vi "IHM_errorManagement.vi"(4 "error out":errorcluster, 6 "Cas no error":T1, 7 "No error Line":string) -> (0 "entrée d'erreur (pas d'erreur)":errorcluster, 2 "Cas IHM":T1, 3 "New line Out":string)   [LabVIEW 2009]
uses:
  Commands/IHM_cases.ctl
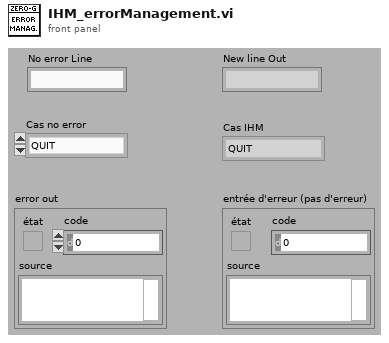
[diagram p1: front panel]
types:
  T1 = typedef "IHM_cases.ctl" = enum16{"QUIT", "INIT IHM", "LOAD CONFIGURATION FILE", "INIT INSTRU", "IHM PROCESS", "CLOSE INSTRU"}
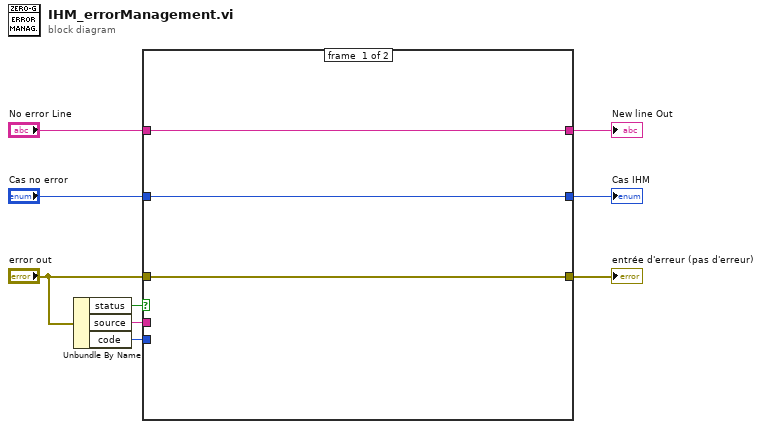
[diagram p0: block diagram]
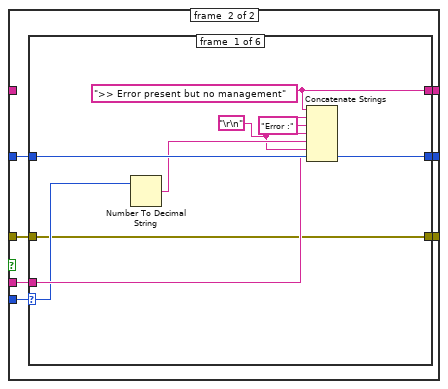
[diagram p2: hidden frame]
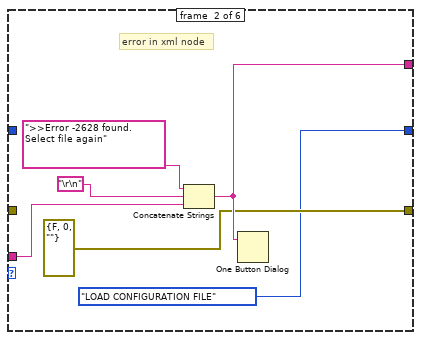
[diagram p3: hidden frame]
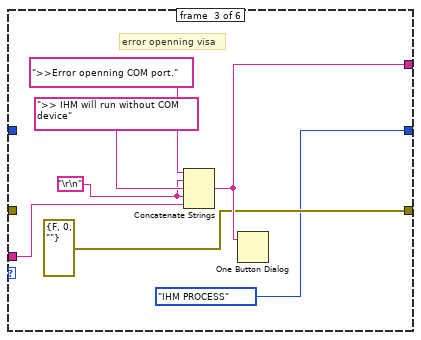
[diagram p4: hidden frame]
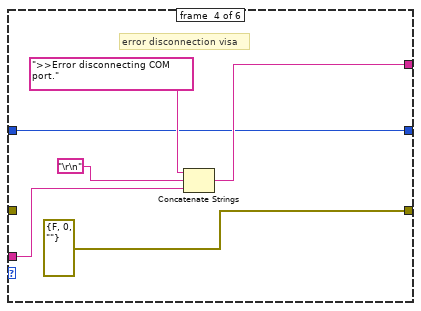
[diagram p5: hidden frame]
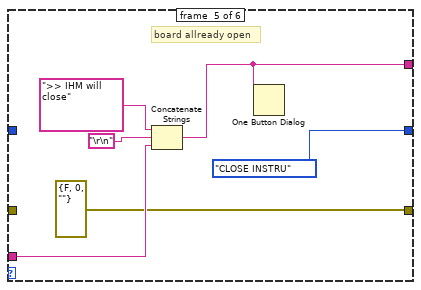
[diagram p6: hidden frame]
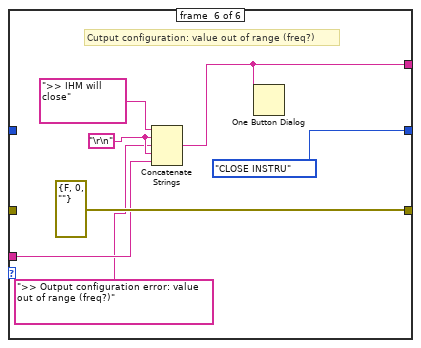
[diagram p7: hidden frame]
diagram:
  n1 = Unbundle By Name("error out") -> ("status"=w8:bool, "source"=w7:string, "code"=w9:i32)
  n2 = case shown="Vrai" w8 {
    tunnel: [w12 w19] -> w4
    tunnel: [w10 w15] -> w5
    tunnel: "error out" -> [w12 w18]
    tunnel: w7 -> [_ w17]
    tunnel: w9 -> [_ w16]
    tunnel: "Cas no error" -> [w11 w13]
    tunnel: [w11 w14] -> w2
    tunnel: "No error Line" -> [w10 _]
    frame #0 {
    }
    frame #1 {
      n3 = case shown="257" w16 {
        selector: w16 -> [w25 _ _ _ _ _]
        tunnel: w18 -> [w20 _ _ _ _ _]
        tunnel: [w20 errorcluster {"status"=FALSE, "code"=0, "source"=""} ("entrée d'erreur (pas d'erreur)") errorcluster {"status"=FALSE, "code"=0, "source"=""} ("entrée d'erreur (pas d'erreur)") errorcluster {"status"=FALSE, "code"=0, "source"=""} ("entrée d'erreur (pas d'erreur)") errorcluster {"status"=FALSE, "code"=0, "source"=""} ("entrée d'erreur (pas d'erreur)") errorcluster {"status"=FALSE, "code"=0, "source"=""} ("entrée d'erreur (pas d'erreur)")] -> w19
        tunnel: [w23 w30 w39 w46 w49 w58] -> w15
        tunnel: w17 -> [w26 w31 w40 w42 w50 w55]
        tunnel: [w27 IHM_cases."LOAD CONFIGURATION FILE" ("Cas IHM") IHM_cases."IHM PROCESS" ("Cas IHM") w41 IHM_cases."CLOSE INSTRU" ("Cas IHM") IHM_cases."CLOSE INSTRU" ("Cas IHM")] -> w14
        tunnel: w13 -> [w27 _ _ w41 _ _]
        frame #0 {
          w22 = "\r\n"
          w23 = ">> Error present but no management" ("New line In")
          n4 = Number To Decimal String(number=w25) -> (decimal integer string=w24:string)  [unwired: 1 in]
          n5 = Concatenate Strings(w23, w22, "Error :" ("chaîne"), w22, w24, w22, w26) -> ()  [unwired: 1 out]
        }
        frame #1 {
          # "error in xml node"
          n6 = Concatenate Strings(">>Error -2628 found. Select file again" ("New line In"), "\r\n", w31) -> (w30:string)
          n7 = One Button Dialog(message=w30) -> ()  [unwired: 1 in, 1 out]
        }
        frame #2 {
          w34 = "\r\n"
          # "error openning visa"
          n8 = Concatenate Strings(">>Error openning COM port." ("New line In"), w34, ">> IHM will run without COM device" ("New line In"), w34, w40) -> (w39:string)
          n9 = One Button Dialog(message=w39) -> ()  [unwired: 1 in, 1 out]
        }
        frame #3 {
          # "error disconnection visa"
          n10 = Concatenate Strings(">>Error disconnecting COM port." ("New line In"), "\r\n", w42) -> (w46:string)
        }
        frame #4 {
          # "board allready open"
          n11 = Concatenate Strings(">> IHM will close" ("New line In"), "\r\n", w50) -> (w49:string)
          n12 = One Button Dialog(message=w49) -> ()  [unwired: 1 in, 1 out]
        }
        frame #5 {
          w54 = "\r\n"
          # "Cutput configuration: value out of range (freq?)"
          n13 = Concatenate Strings(">> IHM will close" ("New line In"), w54, ">> Output configuration error: value out of range (freq?)" ("New line In"), w54, w55) -> (w58:string)
          n14 = One Button Dialog(message=w58) -> ()  [unwired: 1 in, 1 out]
        }
      }
    }
  }
  "New line Out" <- w5
  "Cas IHM" <- w2
  "entrée d'erreur (pas d'erreur)" <- w4
